vi "sequence path locator.vi"(7 "Sequence folder name":string="Sequences", 8 "sequence path":string, 9 "Sequences folder path":path=path "C:/Users/shared/Sequences", 10 "Use absolute sequence path":bool, 11 "platform":u16(ring) items=["Mac", "PC"]) -> (3 "modified path":string)   [LabVIEW 2021]
panel:
  # "(if abs. path not used)"
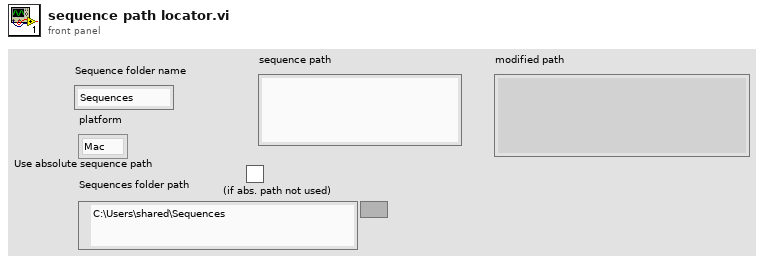
[diagram p1: front panel]
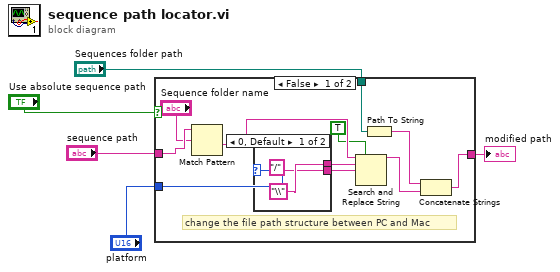
[diagram p0: block diagram]
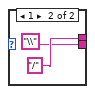
[diagram p2: hidden frame]
diagram:
  n1 = case shown="False" "Use absolute sequence path" {
    tunnel: "sequence path" -> [w16 w21]
    tunnel: [w9 w21] -> w1
    tunnel: "platform" -> [w10 _]
    tunnel: "Sequences folder path" -> [w8 _]
    frame False {
      # "change the file path structure between PC and Mac"
      n2 = Match Pattern(string=w16, regular expression="Sequence folder name") -> (after substring=w11:string)  [unwired: 1 in, 3 out]
      n3 = case shown="0, Default" w10 {
        tunnel: ["\\" "/"] -> w15
        tunnel: ["/" "\\"] -> w14
        frame 0, Default {
        }
        frame 1 {
        }
      }
      n4 = Search and Replace String(replace all?=TRUE ("replace all? (F)"), input string=w11, search string=w15, replace string=w14) -> (result string=w12:string)  [unwired: 4 in, 3 out]
      n5 = Path To String(path=w8) -> (string=w13:string)
      n6 = Concatenate Strings(w13, w12) -> (w9:string)
    }
    frame True {
    }
  }
  "modified path" <- w1
